vi "Izhikevich_primitive_v004.vi"(0 "UDP Network Connection in":refnum<k16>, 1 "b":dbl, 2 "a":dbl, 3 "I":dbl, 5 "c":dbl, 7 "d":dbl, 9 "v(t)":dbl, 11 "error in (no error)":errorcluster, 12 "u(t)":dbl, 13 "Numeric":dbl, 14 "Address selector":i32[](array[numeric])) -> (4 "UDP Network Connection out":refnum<k16>, 6 "v(t+dt)":dbl, 8 "u(t+dt)":dbl, 15 "error out":errorcluster)   [LabVIEW 2019]
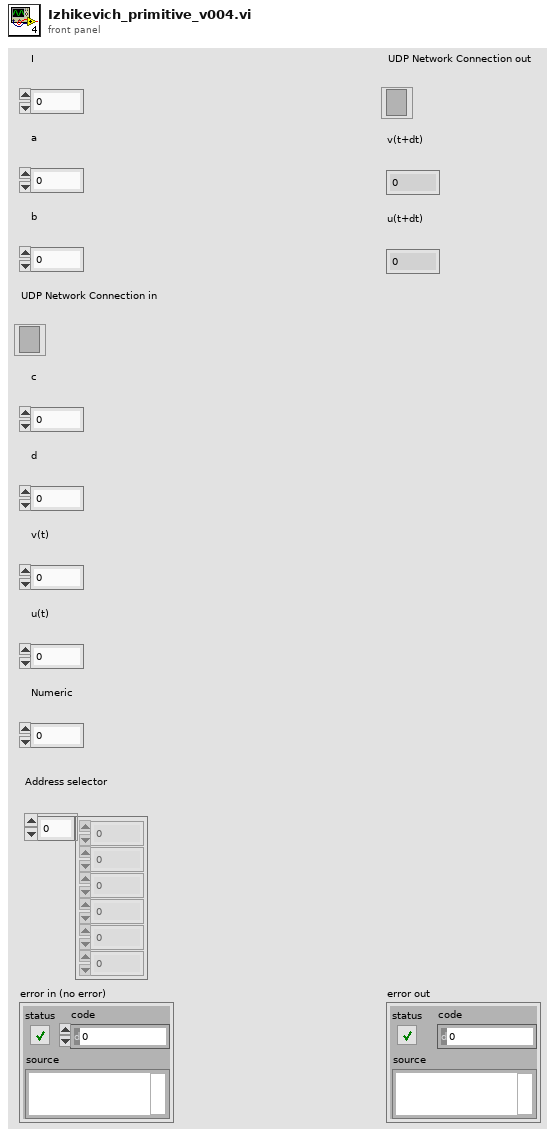
[diagram p1: front panel]
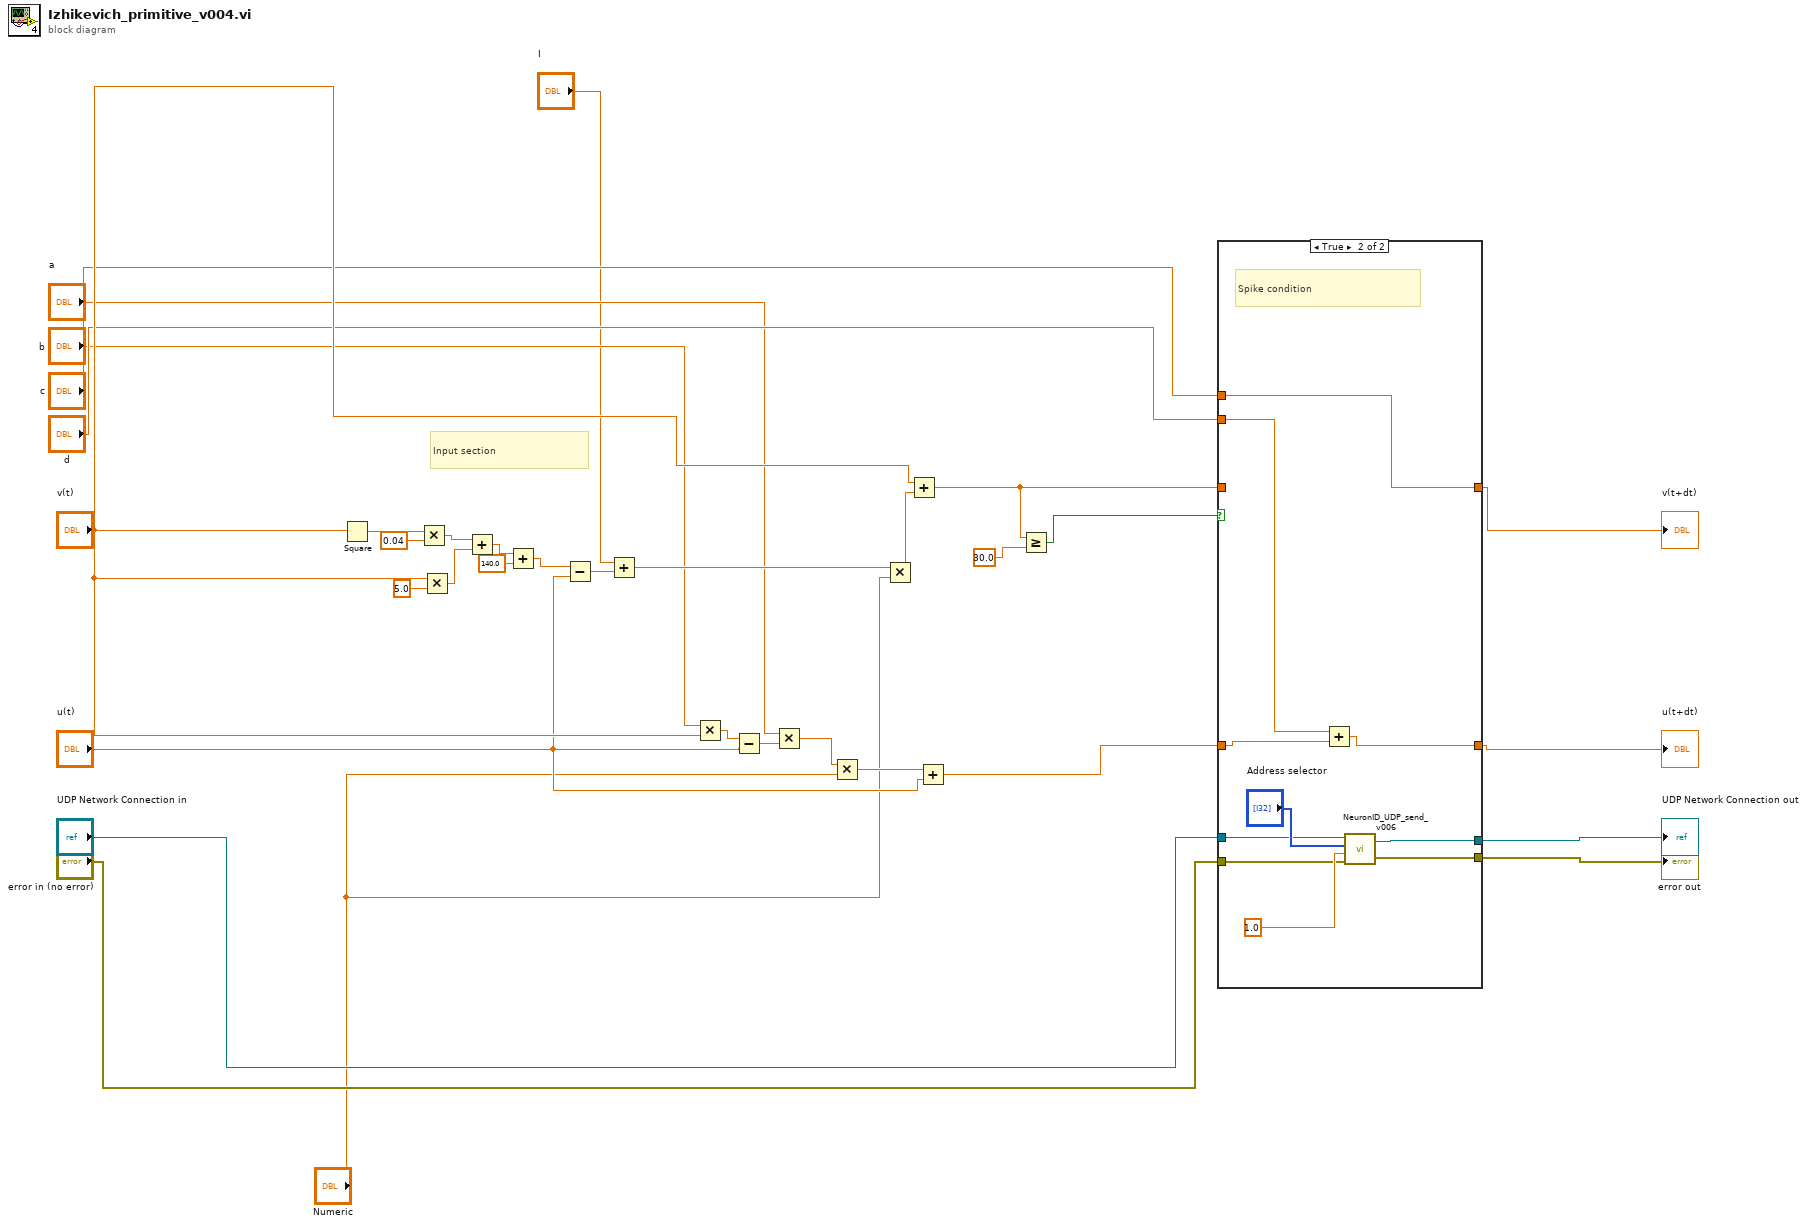
[diagram p0: block diagram]
diagram:
  # "Input section"
  n1 = Square(x="v(t)") -> (x^2=w1:dbl)
  n2 = Multiply(x=w1, y=0.04) -> (x*y=w3:dbl)
  n3 = Multiply(x="v(t)", y=5.0) -> (x*y=w5:dbl)
  n4 = Add(x=w3, y=w5) -> (x+y=w6:dbl)
  n5 = Add(x=w6, y=140.0) -> (x+y=w8:dbl)
  n6 = Subtract(x=w8, y="u(t)") -> (x-y=w9:dbl)
  n7 = Add(x="I", y=w9) -> (x+y=w16:dbl)
  n8 = Multiply(x="b", y="v(t)") -> (x*y=w12:dbl)
  n9 = Subtract(x=w12, y="u(t)") -> (x-y=w13:dbl)
  n10 = Multiply(x="a", y=w13) -> (x*y=w15:dbl)
  n11 = Multiply(x=w15, y="Numeric") -> (x*y=w19:dbl)
  n12 = Multiply(x=w16, y="Numeric") -> (x*y=w18:dbl)
  n13 = Add(x="v(t)", y=w18) -> (x+y=w28:dbl)
  n14 = Add(x=w19, y="u(t)") -> (x+y=w21:dbl)
  n15 = Greater Or Equal?(x=w28, y=30.0) -> (x >= y?=w29:bool)
  n16 = case shown="True" w29 {
    tunnel: [w37 w44] -> w20
    tunnel: w21 -> [w37 w46]
    tunnel: w28 -> [w36 _]
    tunnel: [w36 w47] -> w22
    tunnel: "c" -> [_ w47]
    tunnel: "d" -> [_ w45]
    tunnel: [w35 w42] -> w30
    tunnel: "error in (no error)" -> [w35 w38]
    tunnel: "UDP Network Connection in" -> [w34 w40]
    tunnel: [w34 w43] -> w32
    frame False {
      # "No spike condition"
    }
    frame True {
      # "Spike condition"
      n17 = Add(x=w45, y=w46) -> (x+y=w44:dbl)
      n18 = call "NeuronID_UDP_send_v006.vi"("error in (no error)"=w38, "Neuron ID"=1.0, "Address selector"="Address selector", "UDP Network Connection in"=w40) -> ("error out"=w42:errorcluster, "UDP Network Connection out"=w43:refnum<k16>)
    }
  }
  "UDP Network Connection out" <- w32
  "error out" <- w30
  "v(t+dt)" <- w22
  "u(t+dt)" <- w20
